vi "ConfigUtilities - Initialize Rx Packet Page Panel.vi"(7 "Channels Listbox":refnum<vi>, 8 "error in (no error)":errorcluster, 9 "Channel Paths Property":string, 10 "Channel Names Property":string, 11 "Item Ref in":T1 format="%.0x") -> (0 "error out":errorcluster, 1 "Channel Paths":string[](array[string]), 2 "Channel Names":string[](array[string]), 3 "Item Ref out":T1 format="%.0x")   [LabVIEW 2015, in "UDP-Custom-Device System Explorer.lvlib"]
doc: "Initialize the Rx Channels Section Page Panel."
uses:
  <vilib>/NI Veristand/Custom Device API/Custom Device Item Ref.ctl
  <vilib>/Utility/miscctls.llb/LVRowAndColumnUnsignedTypeDef.ctl
  <vilib>/NI Veristand/Custom Device API/Get Item Property (String Array).vi
  UDP-Custom-Device System Explorer.lvlib
  <vilib>/NI VeriStand/Custom Device API/Custom Device API.lvlib
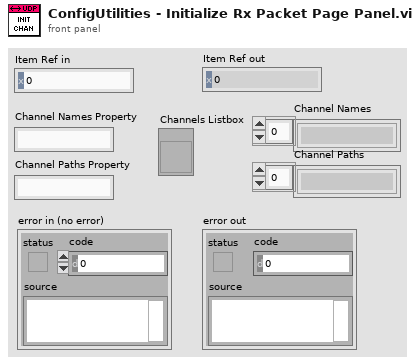
[diagram p1: front panel]
types:
  T1 = typedef "Custom Device API.lvlib/Custom Device Item Ref.ctl" = u64
  T2 = typedef "LVRowAndColumnUnsignedTypeDef.ctl" = cluster{"Row":u32, "Column":u32}
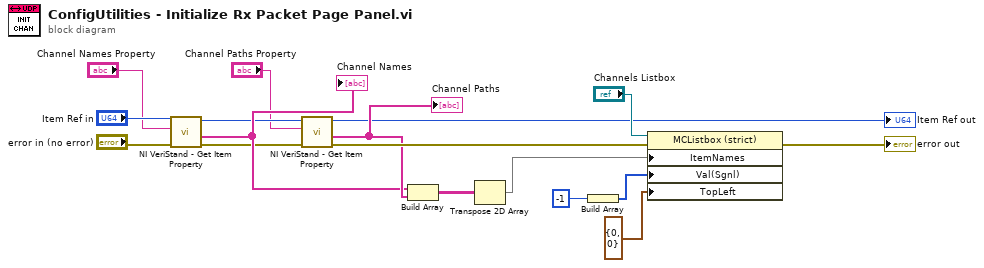
[diagram p0: block diagram]
diagram:
  n1 = call-poly <vilib>:"NI VeriStand - Get Item Property.vi"("error in (no error)"="error in (no error)", "Property Name"="Channel Names Property", "Item Ref in"="Item Ref in") -> ("error out"=w9:errorcluster, "Value"=w12:string[], "Item Ref out"=w8:T1)  [unwired: 5 in, 1 out]
  "Channel Names" <- w12
  n2 = call-poly <vilib>:"NI VeriStand - Get Item Property.vi"("error in (no error)"=w9, "Property Name"="Channel Paths Property", "Item Ref in"=w8) -> ("error out"=w14:errorcluster, "Value"=w13:string[], "Item Ref out"=→"Item Ref out":T1)  [unwired: 5 in, 1 out]
  "Channel Paths" <- w13
  n3 = Build Array(w12, w13) -> (w10:string[][])
  n4 = Transpose 2D Array(2D array=w10) -> (transposed array=w15:string[][])
  n5 = Build Array(-1) -> (w16:i32[])
  n6 = property class="MCListbox (strict)"(reference="Channels Listbox", error in=w14, "ItemNames"=w15, "Val(Sgnl)"=w16, "TopLeft"=T2 {"Row"=0, "Column"=0} ("Top Left Visible Cell")) -> (error out=→"error out":errorcluster)  [unwired: 1 out]
